vi "Waveform_Indexing.vi"(0 "index":i32, 2 "waveform":waveform(dbl)) -> (7 "output waveform":waveform(dbl))   [LabVIEW 2021]
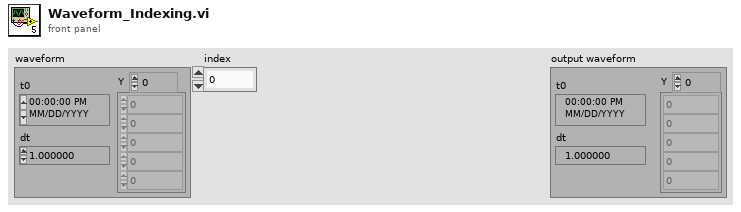
[diagram p1: front panel]
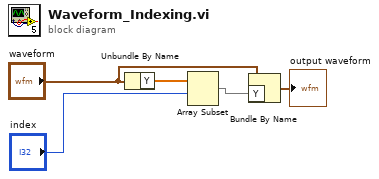
[diagram p0: block diagram]
diagram:
  n1 = Unbundle By Name("waveform") -> ("Y"=w5:dbl[])
  n2 = Array Subset(array=w5, index="index") -> (w4:dbl[])  [unwired: 1 in]
  n3 = Bundle By Name(cluster="waveform", "Y"=w4) -> (→"output waveform":waveform(dbl))
